vi "get_resolution.vi"(8 "error in (no error)":errorcluster, 11 "TrajectoryAK101022Resonance in":refnum<class "TrajectoryAK101022Resonance.lvclass">) -> (0 "error out":errorcluster, 1 "y resolution":i32, 2 "x resolution":i32, 3 "TrajectoryAK101022Resonance out":refnum<class "TrajectoryAK101022Resonance.lvclass">)   [LabVIEW 2010, in "TrajectoryAK101022Resonance.lvclass"]
uses:
  TrajectoryAK101022Resonance.lvclass
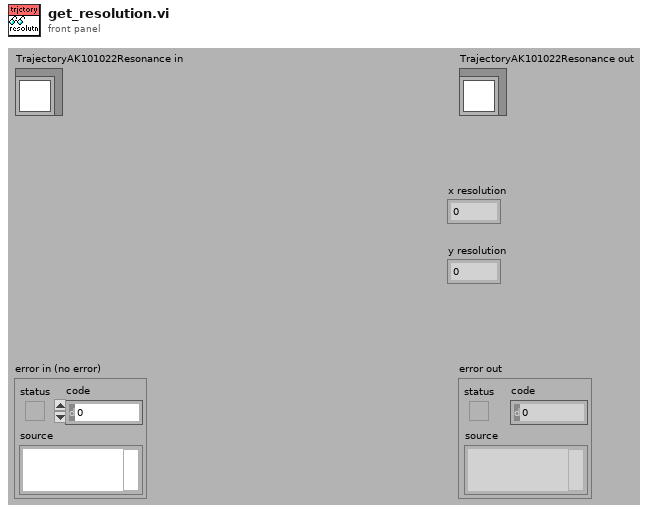
[diagram p1: front panel]
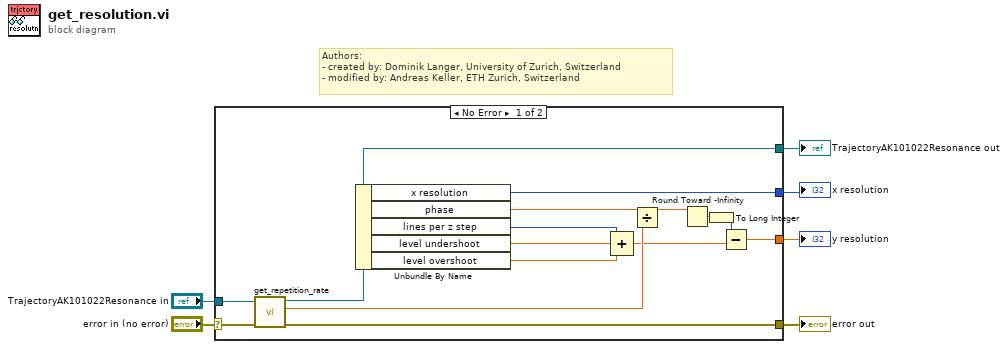
[diagram p0: block diagram]
diagram:
  # "Authors: \n- created by: Dominik Langer, University of Zurich, Switzerland\n- modified by: Andreas Keller, ETH Zurich, Switzerland"
  n1 = case shown="No Error" "error in (no error)" {
    selector: "error in (no error)" -> [w20 w23]
    tunnel: [w19 w23] -> w5
    tunnel: [w17 w22] -> w3
    tunnel: "TrajectoryAK101022Resonance in" -> [w18 w22]
    tunnel: [w21 _] -> w2
    tunnel: [w7 _] -> w1
    frame No Error {
      n2 = call-dynamic "get_repetition_rate.vi"("error in (no error)"=w20, "GenericTrajectory in"=w18) -> ("error out"=w19:errorcluster, "repetition rate"=w15:dbl[unit], "GenericTrajectory out"=w17:refnum<class "TrajectoryAK101022Resonance.lvclass">)  [unwired: 7 in]
      n3 = Unbundle By Name(w17) -> ("x resolution"=w21:i32, "phase"=w16:dbl, "lines per z step"=w12:i32, "level undershoot"=w11:dbl, "level overshoot"=w10:dbl)
      n4 = Compound Arithmetic op=ADD(w12, w11, w10) -> (w9:dbl)
      n5 = Divide(x=w16, y=w15) -> (x/y=w14:dbl[unit])
      n6 = Round Toward -Infinity(1:w14) -> (0:w13:dbl)
      n7 = To Long Integer(number=w13) -> (32bit integer=w8:i32)
      n8 = Subtract(x=w8, y=w9) -> (x-y=w7:dbl)
    }
    frame Error {
    }
  }
  "error out" <- w5
  "TrajectoryAK101022Resonance out" <- w3
  "y resolution" <- w1
  "x resolution" <- w2
